vi "BuildZLUT.vi"(11 "MeasureConfig":T2={"Bead locations"=[{"X"=0, "Y"=0}], "ROI"=200, "Experiment base path"=path "", "Image output subdir"="images", "Output mode"=enum."None", "Traces output subdir"="traces", "QTrk Settings"={"Image width"=150, "Image height"=150, "Number of threads (CPU based)"=-1, "CUDA Device"=-2, "COM Background correction factor"=0.0, "ZLUT MinRadius"=8.0, "ZLUT Radial sample density"=5.0, "ZLUT Angular sample density"=2.0, "ZLUT ROI Coverage"=0.7, "QI Iterations"=1, "QI MinRadius"=2.0, "QI Radial sample density"=5.0, "QI Angular sample density"=2.0, "QI ROI Coverage"=0.7, "QI Angular Step \nIteration Factor"=0.8, "XCOR Profile Length"=1, "XCOR Profile Width"=128, "XCOR Iterations"=32, "Gaussian 2D Fit Iterations"=2, "Gaussian 2D Sigma (pixels)"=3.0, "Downsample"=0}, "Tracking Config"={"Number of steps"=0, "ZLUT stepsize (um)"=0.0, "Z correction factor"=0.0, "Start piezo Z (um)"=0.0, "Pixel size (nm)"=0.0, "2D Localization Type"=enum."Quadrant Interpolation", "Z Command (None)"=enum."Nothing", "Z Piezo scale"=FALSE, "ZLUT Building\nimages per frame"=0, "ZLUT Bias correction planes"=1}, "Experiment Name"="", "Program"={"Commands"=[], "Motor Axis accuracy conditions"={"Magnet Z"=0.0, "Magnet rotation"=0.0, "Camera"={"X"=0.0, "Y"=0.0}, "Piezo XY"={"X"=0.0, "Y"=0.0}, "Piezo Z"=0.0}, "Axis flags"={"Magnet Z"=FALSE, "Magnet rotation"=FALSE, "Camera"={"X"=FALSE, "Y"=FALSE}, "Piezo XY"={"X"=FALSE, "Y"=FALSE}, "Piezo Z"=FALSE}}, "ZLUT"=[], "Camera settings"={"Framerate (Hz)"=60, "Exposure time (us)"=5000, "Image size"={"Width"=1280, "Height"=1024}, "Number of buffers"=30}, "Experiment Script"="", "Max frames in memory"=10000, "Save traces as binary"=FALSE, "Pixel Calibration Gain Image"="camera_calib_gain.bin", "Pixel Calibration Offset Image"="camera_calib_offset.bin", "Use pixel calibration images"=FALSE, "Internal camera settings"="", "Trace write interval"=100} {"QTrk Settings"."QI ROI Coverage" format="%_2g"; "QTrk Settings"."QI MinRadius" format="%.2f"; "QTrk Settings"."QI Angular sample density" format="%.3f"; "QTrk Settings"."QI Radial sample density" format="%.2f"; "QTrk Settings"."ZLUT Radial sample density" format="%.2f"; "QTrk Settings"."ZLUT MinRadius" format="%.2f"}) -> (2 "Is cancelled?":bool, 3 "ZLUT":sgl[][][](array[numeric]))   [LabVIEW 2011]
uses:
  Typedefs/MeasureConfigType.ctl
  Typedefs/MeasureConfigOutputMode.ctl
  qtrk/QTrkLVBinding/QTrkSettings.ctl
  Typedefs/TrackingConfigType.ctl
  qtrk/QTrkLVBinding/QTrkLocalizationType.ctl
  qtrk/QTrkLVBinding/QTrkZCommandType.ctl
  ExperimentProgram/ExperimentProgramType.ctl
  ExperimentProgram/ExProgCommandType.ctl
  ExperimentProgram/ExProgCommandEnumType.ctl
  Motors/MotorAxisEnum.ctl
  Motors/MotorPosType.ctl
  Typedefs/XYf.ctl
  Motors/MotorPosFlagsType.ctl
  Camera/GenericCameraConfigType.ctl
  <vilib>/vision/Image Controls.llb/IMAQ Image.ctl
  Camera/CIGrabControlMsg.ctl
  Camera/CIGrabControlMsgEnum.ctl
  GlobalVariables.vi
panel:
  in  "thread id":i32
  in  "Get debug image?":bool
  out "dbg image":sgl[][](graph)
  in  "Grab Framerate (Hz)":i32=20
  out "Image":T1(plugin-control)
  in  "Check for motor position?":bool=TRUE
  in  "Image available?":bool
  in  "stop capturing":bool
  out "total result count":i32
  out "QTrk result count":i32
  out "Piezo Z":sgl
  in  "Cancel":bool
  out "Frame #":i32
  out "last image grabbed":T1
  out "Total # of steps":i32
  out "Step":i32
  # "Building Z lookup table..."
  # "(used for commands with string parameters)"
  # "-2: Use all devices\n-1: Use best device"
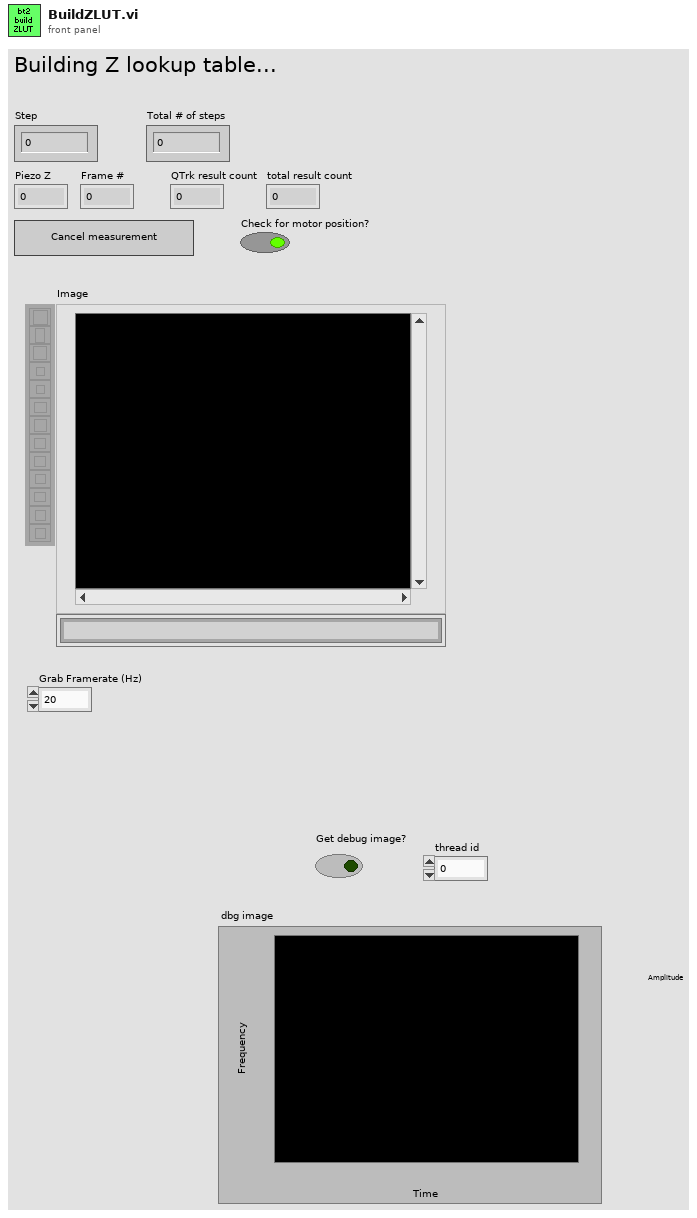
[diagram p1: front panel]
types:
  T1 = typedef "IMAQ Image.ctl" = refnum<image>
  T2 = typedef "MeasureConfigType.ctl" = cluster{"Bead locations":cluster{"X":i32, "Y":i32}[], "ROI":i32, "Experiment base path":path, "Image output subdir":string, "Output mode":T3, "Traces output subdir":string, "QTrk Settings":T4, "Tracking Config":T5, "Experiment Name":string, "Program":T8, "ZLUT":sgl[][][], "Camera settings":T15, "Experiment Script":string, "Max frames in memory":i32, "Save traces as binary":bool, "Pixel Calibration Gain Image":string, "Pixel Calibration Offset Image":string, "Use pixel calibration images":bool, "Internal camera settings":string, "Trace write interval":i32}
  T3 = typedef "MeasureConfigOutputMode.ctl" = enum16{"None", "Track", "SaveImages"}
  T4 = typedef "QTrkSettings.ctl" = cluster{"Image width":i32, "Image height":i32, "Number of threads (CPU based)":i32, "CUDA Device":i32, "COM Background correction factor":sgl, "ZLUT MinRadius":sgl, "ZLUT Radial sample density":sgl, "ZLUT Angular sample density":sgl, "ZLUT ROI Coverage":sgl, "QI Iterations":i32, "QI MinRadius":sgl, "QI Radial sample density":sgl, "QI Angular sample density":sgl, "QI ROI Coverage":sgl, "QI Angular Step \nIteration Factor":sgl, "XCOR Profile Length":i32, "XCOR Profile Width":i32, "XCOR Iterations":i32, "Gaussian 2D Fit Iterations":i32, "Gaussian 2D Sigma (pixels)":sgl, "Downsample":i32}
  T5 = typedef "TrackingConfigType.ctl" = cluster{"Number of steps":i32, "ZLUT stepsize (um)":sgl, "Z correction factor":sgl, "Start piezo Z (um)":sgl, "Pixel size (nm)":sgl, "2D Localization Type":T6, "Z Command (None)":T7, "Z Piezo scale":bool, "ZLUT Building\nimages per frame":i32, "ZLUT Bias correction planes":i32}
  T6 = typedef "QTrkLocalizationType.ctl" = enum16{"Center-of-Mass", "1D Cross-Correlation", "Quadrant Interpolation", "Gaussian 2D MLE", "QI + ZLUTAlign", "ZLUTAlign", "QI + FourierLUT"}
  T7 = typedef "QTrkZCommandType.ctl" = enum16{"Nothing", "ComputeZ", "BuildRadialZLUT", "BuildImageZLUT", "RadialZLUT+ImageZLUT"}
  T8 = typedef "ExperimentProgramType.ctl" = cluster{"Commands":T9[], "Motor Axis accuracy conditions":T12, "Axis flags":T14}
  T9 = typedef "ExProgCommandType.ctl" = cluster{"cmd":T10, "axis":T11, "value/pos":dbl, "speed":dbl, "name":string}
  T10 = typedef "ExProgCommandEnumType.ctl" = enum16{"wait", "move", "event", "idle", "when", "section", "stop"}
  T11 = typedef "MotorAxisEnum.ctl" = enum16{"no axis", "magrot", "magpos", "px", "py", "pz", "camx", "camy"}
  T12 = typedef "MotorPosType.ctl" = cluster{"Magnet Z":dbl, "Magnet rotation":dbl, "Camera":T13, "Piezo XY":T13, "Piezo Z":dbl}
  T13 = typedef "XYf.ctl" = cluster{"X":sgl, "Y":sgl}
  T14 = typedef "MotorPosFlagsType.ctl" = cluster{"Magnet Z":bool, "Magnet rotation":bool, "Camera":cluster{"X":bool, "Y":bool}, "Piezo XY":cluster{"X":bool, "Y":bool}, "Piezo Z":bool}
  T15 = typedef "GenericCameraConfigType.ctl" = cluster{"Framerate (Hz)":i32, "Exposure time (us)":i32, "Image size":cluster{"Width":i32, "Height":i32}, "Number of buffers":i32}
  T16 = typedef "MotorStateType.ctl" = cluster{"Enabled?":bool, "Current Position":T12, "Update counter":i32}
  T17 = typedef "QTrkInstance.ctl" = cluster{"QTrk Pointer":u64}
  T18 = typedef "QTrkComputedSettings.ctl" = cluster{"QTrk Settings":T4, "Derived settings":cluster{"ZLUT Radial Steps":i32, "ZLUT Angular Steps":i32, "ZLUT Max Radius":sgl, "QI Radial Steps":i32, "QI Angular Steps\nPer Quadrant":i32, "QI Max Radius":sgl}}
  T19 = typedef "PixelCalibrationDataType.ctl" = cluster{"Offset image":T1, "Gain image":T1, "Use offset":bool, "Use gain":bool}
  T20 = typedef "CIGrabType.ctl" = refnum<vi>
  T21 = typedef "CmdData_NewFrame.ctl" = cluster{"Buffer Image":T1, "Frame #":i32, "Hardware ROI Index":i32, "Timestamp":dbl, "Type":T22}
  T22 = typedef "CmdEnum_CameraFrameType.ctl" = enum16{"Full", "HardwareROI", "EndGrabMarker"}
  T23 = typedef "CIGrabControlMsg.ctl" = cluster{"Msg":T24}
  T24 = typedef "CIGrabControlMsgEnum.ctl" = enum16{"Stop", "EnableTracking", "DisableTracking"}
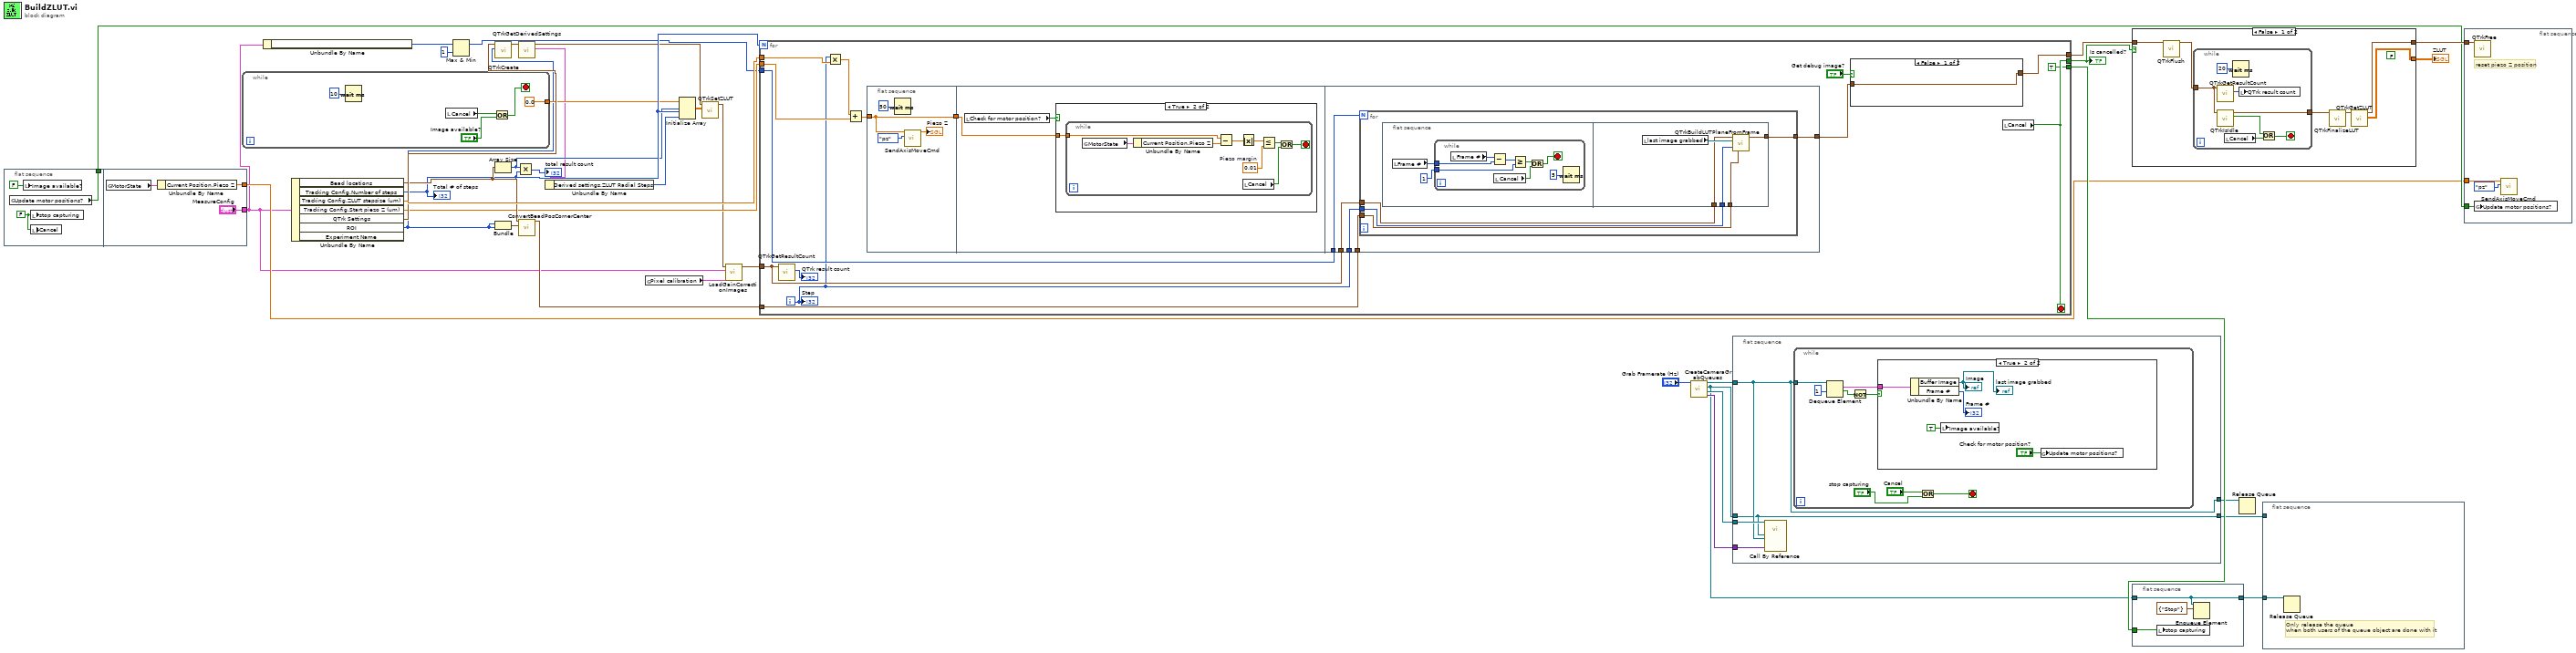
[diagram p0: block diagram]
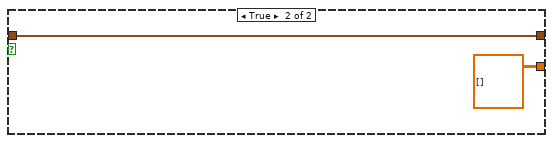
[diagram p3: hidden frame]
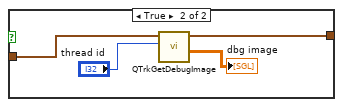
[diagram p4: hidden frame]
diagram:
  n1 = flat-sequence {
    tunnel: [w39] -> w21
    tunnel: ["MeasureConfig"] -> w6
    tunnel: [w42] -> w20
    frame #0 {
      w40 = FALSE ("Cancel")
      n2 = global read "GlobalVariables.vi" "Update motor positions?"() -> (w39:bool)
      n3 = local write "Image available?"(FALSE ("Image available?")) -> ()
      n4 = local write "stop capturing"(w40) -> ()
      n5 = local write "Cancel"(w40) -> ()
    }
    frame #1 {
      n6 = global read "GlobalVariables.vi" "MotorState"() -> (w43:T16)
      n7 = Unbundle By Name(w43) -> ("Current Position.Piezo Z"=w42:dbl)
    }
  }
  n8 = while {
    tunnel: [sgl 0.0 ("element")] -> w26
    stop <- w45 stop-if-true
    n9 = Wait (ms)(milliseconds to wait=u32 10) -> ()  [unwired: 1 out]
    n10 = local read "Cancel"() -> (w47:bool)
    n11 = Or(x=w47, y="Image available?") -> (x .or. y?=w45:bool)
  }
  n12 = Unbundle By Name(w6) -> ("Tracking Config.ZLUT Building\nimages per frame"=w5:i32)
  n13 = Unbundle By Name(w6) -> ("Bead locations"=w35:cluster{"X":i32, "Y":i32}[], "Tracking Config.Number of steps"=w29:i32, "Tracking Config.ZLUT stepsize (um)"=w38:sgl, "Tracking Config.Start piezo Z (um)"=w25:sgl, "QTrk Settings"=w37:T4, "ROI"=w23:i32)  [unwired: 1 out]
  "Total # of steps" <- w29
  n14 = Max & Min(x=w5, y=1) -> (max(x,y)=w3:i32)  [unwired: 1 out]
  n15 = call "QTrkCreate.vi"("ROI"=w23, "QTrk Settings"=w37) -> ("QTrk Instance"=w19:T17)  [unwired: 3 in, 2 out]
  n16 = Array Size(array=w35) -> (size(s)=w24:i32)
  n17 = Bundle("ROI"=w23, "ROI"=w23) -> (w22:cluster{"ROI":i32, "ROI":i32})  [unwired: 1 in]
  n18 = Multiply(x=w24, y=w29) -> (x*y=→"total result count":i32)
  n19 = call "QTrkGetDerivedSettings.vi"("QTrk Instance"=w19) -> ("Derived settings"=w18:T18, "QTrk Instance (out)"=w7:T17)  [unwired: 5 in, 4 out]
  n20 = call "ConvertBeadPosCornerCenter.vi"("ROI Size"=w22, "Center-based bead locations"=w35) -> ("Corner-based bead pos (out)"=w34:cluster{"X":i32, "Y":i32}[])  [unwired: 8 in, 1 out]
  n21 = Unbundle By Name(w18) -> ("Derived settings.ZLUT Radial Steps"=w17:i32)
  n22 = global read "GlobalVariables.vi" "Pixel calibration"() -> (w2:T19)
  n23 = Initialize Array(w26, w24, w29, w17) -> (w36:sgl[][][])
  n24 = call "QTrkSetZLUT.vi"("ZLUT"=w36, "QTrk Instance"=w7) -> ("QTrk Instance"=w16:T17)  [unwired: 8 in, 1 out]
  n25 = call "LoadGainCorrectionImages.vi"("Pixel calibration"=w2, "MeasureConfig"=w6, "QTrk Instance in"=w16) -> ("QTrk Instance out"=w1:T17)  [unwired: 7 in, 1 out]
  n26 = for {
    N: w29 -> [_]
    tunnel: w38 -> [w64]
    tunnel: w25 -> [w62]
    tunnel: w1 -> [w53]
    tunnel: [w55] -> w31
    tunnel: w34 -> [w51]
    tunnel: [w60] -> w30
    tunnel: [TRUE ("stop capturing")] -> w27
    tunnel: w3 -> [w54]
    i -> [w52]
    stop <- w60 stop-if-true
    n27 = call "QTrkGetResultCount.vi"("QTrk Instance"=w53) -> ("result count"=→"QTrk result count":i32)  [unwired: 4 in, 2 out]
    n28 = Multiply(x=w52, y=w64) -> (x*y=w63:sgl)
    n29 = Add(x=w63, y=w62) -> (x+y=w61:sgl)
    n30 = flat-sequence {
      tunnel: w61 -> [w72]
      tunnel: [w72] -> w57
      tunnel: w57 -> [w75]
      tunnel: w54 -> [w90]
      tunnel: w53 -> [w89]
      tunnel: w52 -> [w88]
      tunnel: w51 -> [w87]
      tunnel: [w86] -> w50
      frame #0 {
        n31 = Wait (ms)(milliseconds to wait=u32 50) -> ()  [unwired: 1 out]
        n32 = call "SendAxisMoveCmd.vi"("axis"=MotorAxisEnum."pz", "Position"=w72) -> ("Limited pos"=→"Piezo Z":dbl)  [unwired: 9 in]
      }
      frame #1 {
        n33 = local read "Check for motor position?"() -> (w74:bool)
        n34 = case shown="True" w74 {
          tunnel: w75 -> [_ w76]
          frame False {
          }
          frame True {
            n35 = while {
              tunnel: w76 -> [w82]
              stop <- w83 stop-if-true
              w78 = 0.01  # Piezo margin
              n36 = global read "GlobalVariables.vi" "MotorState"() -> (w85:T16)
              n37 = Unbundle By Name(w85) -> ("Current Position.Piezo Z"=w81:dbl)
              n38 = Subtract(x=w82, y=w81) -> (x-y=w80:dbl)
              n39 = Absolute Value(x=w80) -> (abs(x)=w79:dbl)
              n40 = local read "Cancel"() -> (w84:bool)
              n41 = Less Or Equal?(x=w79, y=w78) -> (x <= y?=w77:bool)
              n42 = Or(x=w77, y=w84) -> (x .or. y?=w83:bool)
            }
          }
        }
      }
      frame #2 {
        n43 = for {
          N: w90 -> [_]
          tunnel: w89 -> [w94]
          tunnel: w88 -> [w93]
          tunnel: w87 -> [w92]
          tunnel: [w91] -> w86
          n44 = flat-sequence {
            tunnel: w94 -> [w108]
            tunnel: w93 -> [w107]
            tunnel: w92 -> [w106]
            tunnel: [w105] -> w91
            frame #0 {
              n45 = local read "Frame #"() -> (w96:i32)
              n46 = while {
                tunnel: w96 -> [w103]
                tunnel: 1 ("Wait frames after motor move") -> [w101]
                stop <- w98 stop-if-true
                n47 = local read "Frame #"() -> (w104:i32)
                n48 = Subtract(x=w104, y=w103) -> (x-y=w102:i32)
                n49 = local read "Cancel"() -> (w97:bool)
                n50 = Greater Or Equal?(x=w102, y=w101) -> (x >= y?=w99:bool)
                n51 = Or(x=w99, y=w97) -> (x .or. y?=w98:bool)
                n52 = Wait (ms)(milliseconds to wait=u32 5) -> ()  [unwired: 1 out]
              }
            }
            frame #1 {
              n53 = local read "last image grabbed"() -> (w109:T1)
              n54 = call "QTrkBuildLUTPlaneFromFrame.vi"("QTrk Instance"=w108, "Image"=w109, "plane"=w107, "ROI Positions (corner-based)"=w106) -> ("QTrk Instance"=w105:T17)  [unwired: 11 in]
            }
          }
        }
      }
    }
    n55 = case shown="False" "Get debug image?" {
      tunnel: w50 -> [w65 w69]
      tunnel: [w65 w68] -> w55
      frame False {
      }
      frame True {
        n56 = call "QTrkGetDebugImage.vi"("id"="thread id", "QTrk Instance"=w69) -> ("data"=→"dbg image":sgl[][], "QTrk Instance (out)"=w68:T17)  [unwired: 7 in, 1 out]
      }
    }
    n57 = local read "Cancel"() -> (w60:bool)
    "Step" <- w52
  }
  "Is cancelled?" <- w30
  n58 = call "CreateCameraGrabQueues.vi"("Framerate (Hz)"="Grab Framerate (Hz)") -> ("Camera state (out)"=w13:variant, "VI refs.Grab"=w14:T20, "GrabControlQueue"=w10:refnum<queue>, "CameraOutQueue"=w12:refnum<queue>)  [unwired: 7 in]
  n59 = flat-sequence {
    tunnel: w14 -> [w113]
    tunnel: w13 -> [w112]
    tunnel: w12 -> [w111]
    tunnel: w10 -> [w110]
    tunnel: [w111] -> w11
    tunnel: [w110] -> w8
    frame #0 {
      n60 = call-by-ref "?"(reference=w113, "Camera data"=w112, "Output Queue"=w111, "GrabControlQueue"=w110) -> ()  [unwired: 9 in, 3 out]
      n61 = while {
        tunnel: w111 -> [w114]
        stop <- w119 stop-if-true
        n62 = Dequeue Element(queue=w114, timeout in ms (-1)=1) -> (element=w117:T21, timed out?=w116:bool)  [unwired: 1 in, 2 out]
        n63 = Not(x=w116) -> (.not. x?=w115:bool)
        n64 = case shown="True" w115 {
          tunnel: w117 -> [_ w126]
          frame False {
          }
          frame True {
            n65 = Unbundle By Name(w126) -> ("Buffer Image"=→"last image grabbed" →"Image":T1, "Frame #"=→"Frame #":i32)
            n66 = local write "Image available?"(TRUE ("Image available?")) -> ()
            n67 = global write "GlobalVariables.vi" "Update motor positions?"("Check for motor position?") -> ()
          }
        }
        n68 = Or(x="Cancel", y="stop capturing") -> (x .or. y?=w119:bool)
      }
    }
  }
  n69 = case shown="False" w30 {
    tunnel: [w132 sgl[][][] [] ("zlut")] -> w33
    tunnel: [w129 w141] -> w32
    tunnel: w31 -> [w131 w141]
    frame False {
      (unwired) FALSE ("Send UI update event? (T)")
      n70 = call "QTrkFlush.vi"("QTrk Instance"=w131) -> ("QTrk Instance (out)"=w130:T17)  [unwired: 9 in, 1 out]
      n71 = while {
        tunnel: w130 -> [w137]
        tunnel: [w139] -> w128
        stop <- w133 stop-if-true
        n72 = call "QTrkGetResultCount.vi"("QTrk Instance"=w137) -> ("result count"=w136:i32)  [unwired: 4 in, 2 out]
        n73 = call "QTrkIsIdle.vi"("QTrk Instance"=w137) -> ("Currently idle?"=w134:bool, "QTrk Instance (out)"=w139:T17)  [unwired: 8 in, 1 out]
        n74 = local read "Cancel"() -> (w135:bool)
        n75 = Wait (ms)(milliseconds to wait=u32 20) -> ()  [unwired: 1 out]
        n76 = local write "QTrk result count"(w136) -> ()
        n77 = Or(x=w134, y=w135) -> (x .or. y?=w133:bool)
      }
      n78 = call "QTrkFinalizeLUT.vi"("QTrk Instance"=w128) -> ("QTrk Instance"=w127:T17)  [unwired: 5 in, 1 out]
      n79 = call "QTrkGetZLUT.vi"("QTrk Instance (in)"=w127) -> ("zlut"=w132:sgl[][][], "QTrk Instance"=w129:T17)  [unwired: 8 in, 1 out]
    }
    frame True {
    }
  }
  "ZLUT" <- w33
  n80 = flat-sequence {
    tunnel: w27 -> [w144]
    tunnel: w10 -> [w142]
    tunnel: [w142] -> w9
    frame #0 {
      n81 = local write "stop capturing"(w144) -> ()
      n82 = Enqueue Element(queue=w142, element=T23 {"Msg"=enum."Stop"}) -> ()  [unwired: 2 in, 3 out]
    }
  }
  n83 = Release Queue(queue=w11) -> ()  [unwired: 2 in, 3 out]
  n84 = flat-sequence {
    tunnel: w9 -> [w145]
    tunnel: w8 -> [_]
    frame #0 {
      # "Only release the queue\nwhen both users of the queue object are done with it"
      n85 = Release Queue(queue=w145) -> ()  [unwired: 2 in, 3 out]
    }
  }
  n86 = flat-sequence {
    tunnel: w32 -> [w149]
    tunnel: w20 -> [w147]
    tunnel: w21 -> [w148]
    frame #0 {
      # "reset piezo Z position"
      n87 = call "QTrkFree.vi"("QTrk Instance"=w149) -> ()  [unwired: 6 in, 1 out]
      n88 = global write "GlobalVariables.vi" "Update motor positions?"(w148) -> ()
      n89 = call "SendAxisMoveCmd.vi"("axis"=MotorAxisEnum."pz", "Position"=w147) -> ()  [unwired: 9 in, 1 out]
    }
  }
